vi "Create.vi"(8 "error in (no error)":errorcluster) -> (0 "error out":errorcluster, 3 "Controller out":refnum<class "Controller.lvclass">)   [LabVIEW 2020, in "Container.lvlib" / "Controller.lvclass"]
uses:
  Controller.lvclass
  Controller.lvclass/Controller.ctl
  Model/Model.lvclass
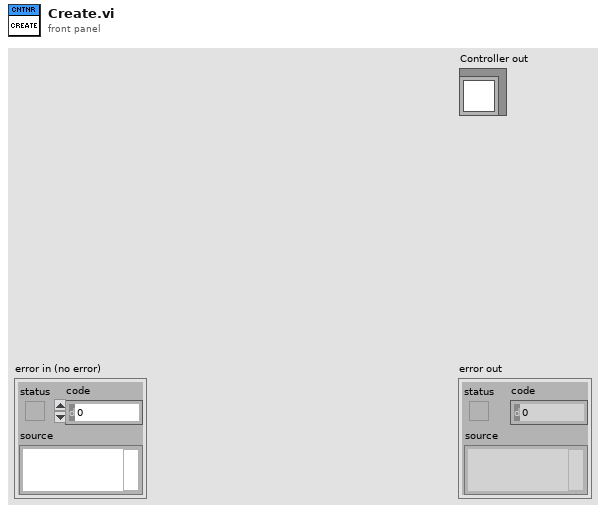
[diagram p1: front panel]
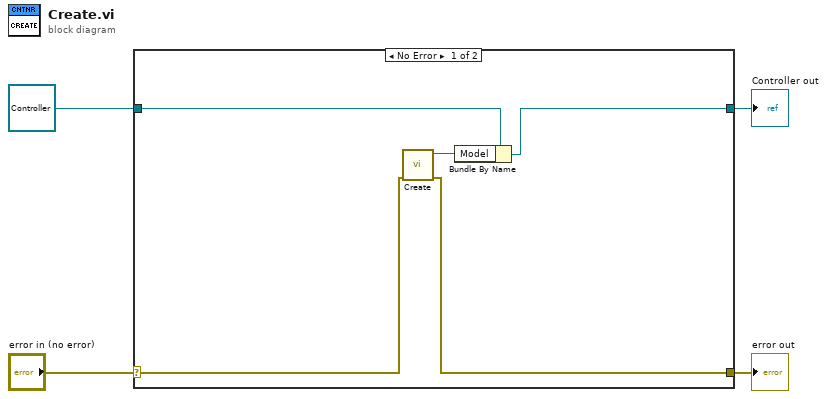
[diagram p0: block diagram]
diagram:
  n1 = case shown="No Error" "error in (no error)" {
    selector: "error in (no error)" -> [w7 w11]
    tunnel: [w5 w11] -> w3
    tunnel: [w6 w10] -> w2
    tunnel: refnum<class "Controller.lvclass"> refnum ("Controller in") -> [w9 w10]
    frame No Error {
      n2 = call "Create.vi"("error in (no error)"=w7) -> ("error out"=w5:errorcluster, "Model out"=w8:refnum<class "Model.lvclass">)  [unwired: 9 in]
      n3 = Bundle By Name(cluster=w9, "Model"=w8) -> (w6:refnum<class "Controller.lvclass">)
    }
    frame Error {
    }
  }
  "error out" <- w3
  "Controller out" <- w2
